vi "Data Generator and Transmitter.vi"   [LabVIEW 2016]
uses:
  <vilib>/Utility/file.llb/Write Delimited Spreadsheet (DBL).vi
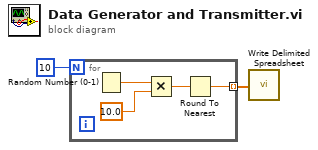
[diagram p0: block diagram]
diagram:
  n1 = for {
    N: 10 -> [_]
    tunnel: [w3] -> w1 mode=indexing
    n2 = Random Number (0-1)() -> (number: 0 to 1=w6:dbl)
    n3 = Multiply(x=w6, y=10.0) -> (x*y=w4:dbl)
    n4 = Round To Nearest(number=w4) -> (nearest integer value=w3:dbl)
  }
  n5 = call-poly <vilib>:"Write Delimited Spreadsheet.vi"("1D data"=w1) -> ()  [unwired: 13 in, 2 out]
